vi "PSAE_VCH_Update VCH List.vi"(8 "Error In (no error)":errorcluster, 10 "VCH":T1, 11 "VCH Ref":refnum<vi>) -> (0 "Error Out":errorcluster)   [LabVIEW 2016]
uses:
  VCH/Private/Ctrls/PSVCH_VCH Info.ctl
panel:
  # "Data Out"
  # "Data In"
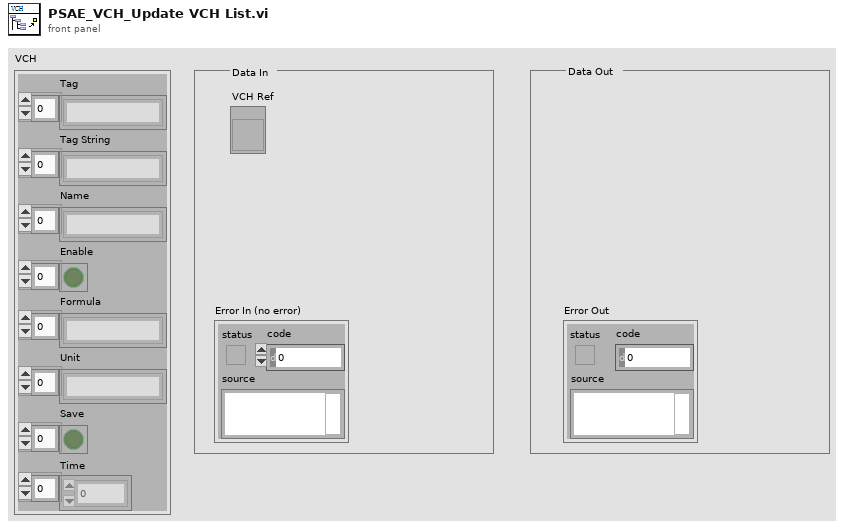
[diagram p1: front panel]
types:
  T1 = typedef "PSVCH_VCH Info.ctl" = cluster{"Tag":string[], "Tag String":string[], "Name":string[], "Enable":bool[], "Formula":string[], "Unit":string[], "Save":bool[], "Time":i64[]}
  T2 = cluster{"Left Cell String":string, "Child Text":string[], "Child Tag":string, "Item Indent":i32, "Child Only?":bool, "Glyph Index":i32}
  T3 = cluster{"Left Cell String":string, "Child Text":string[], "Child Tag":string, "Item Indent":i32, "Child Only?":bool, "Glyph Index":i32}[]
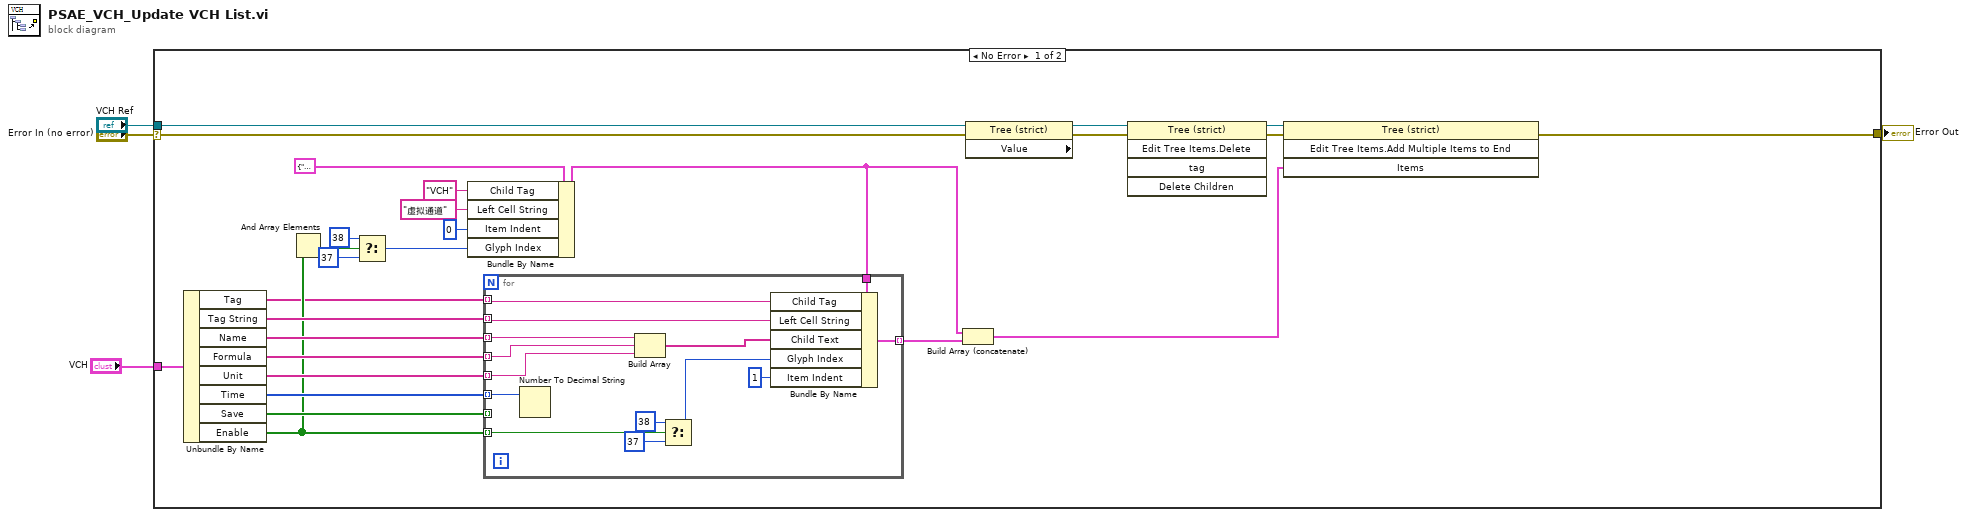
[diagram p0: block diagram]
diagram:
  n1 = case shown="No Error" "Error In (no error)" {
    selector: "Error In (no error)" -> [w9 w46]
    tunnel: "VCH Ref" -> [w10 _]
    tunnel: [w5 w46] -> w3
    tunnel: "VCH" -> [w29 _]
    frame No Error {
      n2 = Unbundle By Name(w29) -> ("Tag"=w6:string[], "Tag String"=w28:string[], "Name"=w27:string[], "Formula"=w24:string[], "Unit"=w25:string[], "Time"=w23:i64[], "Save"=w26:bool[], "Enable"=w15:bool[])
      n3 = And Array Elements(Boolean array=w15) -> (logical AND=w12:bool)
      n4 = Select(t=38 ("Glyph Index"), s=w12, f=37 ("Glyph Index")) -> (s? t:f=w11:i32)
      n5 = Bundle By Name(cluster=T2 {"Left Cell String"="", "Child Text"=[], "Child Tag"="", "Item Indent"=0, "Child Only?"=FALSE, "Glyph Index"=0} ("Item"), "Child Tag"="VCH", "Left Cell String"="虚拟通道", "Item Indent"=0, "Glyph Index"=w11) -> (w20:T2)
      n6 = for {
        tunnel: w6 -> [w43] mode=indexing
        tunnel: w28 -> [w42] mode=indexing
        tunnel: w27 -> [w41] mode=indexing
        tunnel: w24 -> [w40] mode=indexing
        tunnel: w25 -> [w33] mode=indexing
        tunnel: w26 -> [_] mode=indexing
        tunnel: w15 -> [w38] mode=indexing
        tunnel: w20 -> [w45]
        tunnel: [w44] -> w22 mode=indexing
        tunnel: w23 -> [w34] mode=indexing
        n7 = Number To Decimal String(number=w34) -> ()  [unwired: 1 in, 1 out]
        n8 = Build Array(w41, w40, w33) -> (w39:string[])
        n9 = Select(t=38 ("Glyph Index"), s=w38, f=37 ("Glyph Index")) -> (s? t:f=w35:i32)
        n10 = Bundle By Name(cluster=w45, "Child Tag"=w43, "Left Cell String"=w42, "Child Text"=w39, "Glyph Index"=w35, "Item Indent"=1) -> (w44:T2)
      }
      n11 = Build Array (concatenate)(w20, w22) -> (w19:T3)
      n12 = property class="Tree (strict)" props=["Value"](reference=w10, error in=w9) -> (reference out=w7:refnum<vi>, error out=w8:errorcluster)  [unwired: 1 out]
      n13 = invoke class="Tree (strict)" method="Edit Tree Items.Delete"(reference=w7, error in=w8) -> (reference out=w30:refnum<vi>, error out=w31:errorcluster)  [unwired: 3 in, 3 out]
      n14 = invoke class="Tree (strict)" method="Edit Tree Items.Add Multiple Items to End"(reference=w30, error in=w31, "Items"=w19) -> (error out=w5:errorcluster)  [unwired: 1 in, 3 out]
    }
    frame Error {
    }
  }
  "Error Out" <- w3
